vi "Lab Panel V5.24.1.vi"() -> ()   [LabVIEW 2013] (continued)
                n201 = Unbundle(w203) -> ("id1"=→"LAB01-TP":bool, "id2"=→"LAB02-TP":bool, "id3"=→"LAB03-TP":bool, "id4"=→"LAB04-TP":bool, "id5"=→"LAB05-TP":bool)
                n202 = local read "TEMP LA05"() -> (w211:T9)
                n203 = local read "TEMP LA04"() -> (w218:T9)
                n204 = local read "TEMP LA02"() -> (w232:T9)
                n205 = local read "TEMP LA03"() -> (w225:T9)
                n206 = local read "TEMP LA01"() -> (w239:T9)
                n207 = Bundle(cluster=w225, "TL-1"=w223, "TN-1"=w222, "TL-2"=w221, "TN-2"=w220) -> (w224:T9)  [unwired: 4 in]
                n208 = Bundle(cluster=w239, "TL-1"=w238, "TN-1"=w237, "TL-2"=w236, "TN-2"=w235) -> (w234:T9)  [unwired: 4 in]
                n209 = Bundle(cluster=w232, "TL-1"=w230, "TN-1"=w229, "TL-2"=w228, "TN-2"=w227) -> (w231:T9)  [unwired: 4 in]
                n210 = Bundle(cluster=w218, "TL-1"=w217, "TN-1"=w216, "TL-2"=w215, "TN-2"=w214) -> (w213:T9)  [unwired: 4 in]
                n211 = Bundle(cluster=w211, "TL-1"=w210, "TN-1"=w209, "TL-2"=w208, "TN-2"=w207) -> (w206:T9)  [unwired: 4 in]
                n212 = local write "TEMP LA03"(w224) -> ()
                n213 = local write "TEMP LA01"(w234) -> ()
                n214 = local write "TEMP LA02"(w231) -> ()
                n215 = local write "TEMP LA05"(w206) -> ()
                n216 = local write "TEMP LA04"(w213) -> ()
              }
            }
            frame #2 {
              w253 = 0
              n217 = local read "LAB01 TEMP"() -> (w255:T12)
              n218 = local read "SIG LAB01-2"() -> (w250:T2)
              n219 = Unbundle By Name(w255) -> ("T1 Live"=w248:dbl, "T1 Neut"=w247:dbl, "T2 Live"=w246:dbl, "T2 Neut"=w245:dbl)  [unwired: 2 out]
              n220 = local read "SIG LAB01-1"() -> (w252:T2)
              n221 = local read "TEMP LA01"() -> (w256:T9)
              n222 = Bundle By Name(cluster=w256, "TL-1"=w248, "TN-1"=w247, "TL-2"=w246, "TN-2"=w245, "TL -1COUNT"=w253, "TN-1 COUNT"=w253, "TL-2 COUNT"=w253, "TN-2 COUNT"=w253) -> (w254:T9)
              n223 = Bundle(cluster=w252, "Tmp Live"=w248, "Tmp Neut"=w247) -> (w251:T2)  [unwired: 3 in]
              n224 = Bundle(cluster=w250, "Tmp Live"=w246, "Tmp Neut"=w245) -> (w249:T2)  [unwired: 3 in]
              n225 = local write "SIG LAB01-2"(w249) -> ()
              n226 = local write "SIG LAB01-1"(w251) -> ()
              n227 = local write "TEMP LA01"(w254) -> ()
            }
            frame #3 {
              w265 = 0
              n228 = local read "LAB02 TEMP"() -> (w267:T12)
              n229 = Unbundle By Name(w267) -> ("T1 Live"=w260:dbl, "T1 Neut"=w259:dbl, "T2 Live"=w258:dbl, "T2 Neut"=w257:dbl)  [unwired: 2 out]
              n230 = local read "SIG LAB02-1"() -> (w264:T2)
              n231 = local read "SIG LAB02-2"() -> (w263:T2)
              n232 = local read "TEMP LA02"() -> (w268:T9)
              n233 = Bundle By Name(cluster=w268, "TL-1"=w260, "TN-1"=w259, "TL-2"=w258, "TN-2"=w257, "TL -1COUNT"=w265, "TN-1 COUNT"=w265, "TL-2 COUNT"=w265, "TN-2 COUNT"=w265) -> (w266:T9)
              n234 = Bundle(cluster=w263, "Tmp Live"=w258, "Tmp Neut"=w257) -> (w261:T2)  [unwired: 3 in]
              n235 = Bundle(cluster=w264, "Tmp Live"=w260, "Tmp Neut"=w259) -> (w262:T2)  [unwired: 3 in]
              n236 = local write "TEMP LA02"(w266) -> ()
              n237 = local write "SIG LAB02-1"(w262) -> ()
              n238 = local write "SIG LAB02-2"(w261) -> ()
            }
            frame #4 {
              w277 = 0
              n239 = local read "LAB03 TEMP"() -> (w279:T12)
              n240 = Unbundle By Name(w279) -> ("T1 Live"=w272:dbl, "T1 Neut"=w271:dbl, "T2 Live"=w270:dbl, "T2 Neut"=w269:dbl)  [unwired: 2 out]
              n241 = local read "SIG LAB03-1"() -> (w276:T2)
              n242 = local read "SIG LAB03-2"() -> (w275:T2)
              n243 = local read "TEMP LA03"() -> (w280:T9)
              n244 = Bundle By Name(cluster=w280, "TL-1"=w272, "TN-1"=w271, "TL-2"=w270, "TN-2"=w269, "TL -1COUNT"=w277, "TN-1 COUNT"=w277, "TL-2 COUNT"=w277, "TN-2 COUNT"=w277) -> (w278:T9)
              n245 = Bundle(cluster=w275, "Tmp Live"=w270, "Tmp Neut"=w269) -> (w273:T2)  [unwired: 3 in]
              n246 = Bundle(cluster=w276, "Tmp Live"=w272, "Tmp Neut"=w271) -> (w274:T2)  [unwired: 3 in]
              n247 = local write "TEMP LA03"(w278) -> ()
              n248 = local write "SIG LAB03-2"(w273) -> ()
              n249 = local write "SIG LAB03-1"(w274) -> ()
            }
            frame #5 {
              w289 = 0
              n250 = local read "LAB04 TEMP"() -> (w291:T12)
              n251 = Unbundle By Name(w291) -> ("T1 Live"=w284:dbl, "T1 Neut"=w283:dbl, "T2 Live"=w282:dbl, "T2 Neut"=w281:dbl)  [unwired: 2 out]
              n252 = local read "SIG LAB04-2"() -> (w287:T2)
              n253 = local read "SIG LAB04-1"() -> (w288:T2)
              n254 = local read "TEMP LA04"() -> (w292:T9)
              n255 = Bundle By Name(cluster=w292, "TL-1"=w284, "TN-1"=w283, "TL-2"=w282, "TN-2"=w281, "TL -1COUNT"=w289, "TN-1 COUNT"=w289, "TL-2 COUNT"=w289, "TN-2 COUNT"=w289) -> (w290:T9)
              n256 = Bundle(cluster=w287, "Tmp Live"=w282, "Tmp Neut"=w281) -> (w285:T2)  [unwired: 3 in]
              n257 = Bundle(cluster=w288, "Tmp Live"=w284, "Tmp Neut"=w283) -> (w286:T2)  [unwired: 3 in]
              n258 = local write "SIG LAB04-2"(w285) -> ()
              n259 = local write "TEMP LA04"(w290) -> ()
              n260 = local write "SIG LAB04-1"(w286) -> ()
            }
            frame #6 {
              w301 = 0
              n261 = local read "LAB05 TEMP"() -> (w303:T12)
              n262 = Unbundle By Name(w303) -> ("T1 Live"=w296:dbl, "T1 Neut"=w295:dbl, "T2 Live"=w294:dbl, "T2 Neut"=w293:dbl)  [unwired: 2 out]
              n263 = local read "SIG LAB05-2"() -> (w299:T2)
              n264 = local read "SIG LAB05-1"() -> (w300:T2)
              n265 = local read "TEMP LA05"() -> (w304:T9)
              n266 = Bundle By Name(cluster=w304, "TL-1"=w296, "TN-1"=w295, "TL-2"=w294, "TN-2"=w293, "TL -1COUNT"=w301, "TN-1 COUNT"=w301, "TL-2 COUNT"=w301, "TN-2 COUNT"=w301) -> (w302:T9)
              n267 = Bundle(cluster=w299, "Tmp Live"=w294, "Tmp Neut"=w293) -> (w297:T2)  [unwired: 3 in]
              n268 = Bundle(cluster=w300, "Tmp Live"=w296, "Tmp Neut"=w295) -> (w298:T2)  [unwired: 3 in]
              n269 = local write "SIG LAB05-2"(w297) -> ()
              n270 = local write "SIG LAB05-1"(w298) -> ()
              n271 = local write "TEMP LA05"(w302) -> ()
            }
          }
        }
        frame #9 {
          # "enable front panel, all settings done"
          n272 = property on="Tab Control 2" class="TabCtl (strict)"("DisabledEnum"=T16."Enabled" ("Disabled")) -> ()  [unwired: 2 in, 2 out]
          n273 = property on="Tab Control 2" class="TabCtl (strict)"("Value"=0) -> ()  [unwired: 2 in, 2 out]
        }
        frame #10 {
          n274 = property on="Tab Control 2" class="TabCtl (strict)"("Value"=0) -> ()  [unwired: 2 in, 2 out]
        }
      }
    }
    frame #2 {
      n275 = node-c288("loop  delay(mS)") -> (w310:T18)  [unwired: 3 in]
      n276 = timed-loop {
        timing: w310 -> [_]
        timing-out: [_] -> w309
        i -> [w336]
        stop <- w313 stop-if-true
        n277 = node-c288() -> ()  [unwired: 1 in, 1 out]
        n278 = local read "Resets Done"() -> (w315:dbl)
        n279 = Greater?(x=w315, y=50) -> (0:w311:bool)
        n280 = local read "SELECT LAB05-2"() -> (w316:T3)
        n281 = local read "SELECT LAB05-1"() -> (w317:T3)
        n282 = local read "SELECT LAB04-2"() -> (w318:T3)
        n283 = local read "SELECT LAB03-1"() -> (w321:T3)
        n284 = Or(x=w311, y="stop") -> (x .or. y?=w313:bool)
        n285 = local read "SELECT LAB02-2"() -> (w322:T3)
        n286 = local read "SELECT LAB01-1"() -> (w325:T3)
        n287 = local read "SELECT LAB03-2"() -> (w320:T3)
        n288 = local read "SELECT LAB01-2"() -> (w324:T3)
        n289 = local read "SELECT LAB04-1"() -> (w319:T3)
        n290 = local read "SELECT LAB02-1"() -> (w323:T3)
        n291 = local read "run lab03-2"() -> (w330:bool)
        n292 = local read "run lab04-1"() -> (w329:bool)
        n293 = local read "run lab05-1"() -> (w327:bool)
        n294 = local read "run lab04-2"() -> (w328:bool)
        n295 = local read "run lab05-2"() -> (w326:bool)
        n296 = local read "run lab03-1"() -> (w331:bool)
        n297 = local read "run lab02-2"() -> (w332:bool)
        n298 = local read "run lab02-1"() -> (w333:bool)
        n299 = local read "run lab01-1"() -> (w335:bool)
        n300 = local read "run lab01-2"() -> (w334:bool)
        n301 = global write "Global display 1.vi" "stop disp"(w313) -> ()
        n302 = stacked-sequence {
          seq-local: [_ w402 _ _ _ _ _ _ _ _ _ _ _ _ _ _ _ _ _ _ _ _ _ _] -> [_ _ _ _ _ w2503 _ _ _ _ _ _ _ _ _ _ _ _ _ _ _ _ _ _]
          seq-local: [_ w401 _ _ _ _ _ _ _ _ _ _ _ _ _ _ _ _ _ _ _ _ _ _] -> [_ _ _ _ _ w2502 _ _ _ _ _ _ _ _ _ _ _ _ _ _ _ _ _ _]
          seq-local: [_ w388 _ _ _ _ _ _ _ _ _ _ _ _ _ _ _ _ _ _ _ _ _ _] -> [_ _ _ _ _ w2501 _ _ _ _ _ _ _ _ _ _ _ _ _ _ _ _ _ _]
          seq-local: [_ w387 _ _ _ _ _ _ _ _ _ _ _ _ _ _ _ _ _ _ _ _ _ _] -> [_ _ _ _ _ w2500 _ _ _ _ _ _ _ _ _ _ _ _ _ _ _ _ _ _]
          seq-local: [_ w386 _ _ _ _ _ _ _ _ _ _ _ _ _ _ _ _ _ _ _ _ _ _] -> [_ _ _ _ _ w2499 _ _ _ _ _ _ _ _ _ _ _ _ _ _ _ _ _ _]
          seq-local: [_ w385 _ _ _ _ _ _ _ _ _ _ _ _ _ _ _ _ _ _ _ _ _ _] -> [_ _ _ _ _ w2498 _ _ _ _ _ _ _ _ _ _ _ _ _ _ _ _ _ _]
          seq-local: [_ w384 _ _ _ _ _ _ _ _ _ _ _ _ _ _ _ _ _ _ _ _ _ _] -> [_ _ _ _ _ w2497 _ _ _ _ _ _ _ _ _ _ _ _ _ _ _ _ _ _]
          seq-local: [_ w383 _ _ _ _ _ _ _ _ _ _ _ _ _ _ _ _ _ _ _ _ _ _] -> [_ _ _ _ _ w2496 _ _ _ _ _ _ _ _ _ _ _ _ _ _ _ _ _ _]
          seq-local: [_ w382 _ _ _ _ _ _ _ _ _ _ _ _ _ _ _ _ _ _ _ _ _ _] -> [_ _ _ _ _ w2495 _ _ _ _ _ _ _ _ _ _ _ _ _ _ _ _ _ _]
          seq-local: [_ w381 _ _ _ _ _ _ _ _ _ _ _ _ _ _ _ _ _ _ _ _ _ _] -> [_ _ _ _ _ w2494 _ _ _ _ _ _ _ _ _ _ _ _ _ _ _ _ _ _]
          seq-local: [_ _ _ _ _ _ _ _ _ _ _ w3626 _ _ _ _ _ _ _ _ _ _ _ _] -> [_ _ _ _ _ _ _ _ _ _ _ _ w3647 _ _ _ _ _ _ _ _ _ _ _]
          tunnel: w335 -> [_ _ w418 w666 w2093 w2523 w2838 w3325 _ _ _ _ _ w3929 _ w4886 _ _ w5173 w5476 w5657 _ _ _]
          tunnel: w334 -> [_ _ w417 w664 w2092 w2522 w2839 w3324 _ _ _ _ _ w3928 _ w4884 _ _ w5172 w5475 w5655 _ _ _]
          tunnel: w333 -> [_ _ w416 w662 w2091 w2521 w2837 w3323 _ _ _ _ _ w3927 _ w4882 _ _ w5171 w5474 w5654 _ _ _]
          tunnel: w332 -> [_ _ w415 w660 w2090 w2520 w2836 w3322 _ _ _ _ _ w3926 _ w4880 _ _ w5170 w5473 w5653 _ _ _]
          tunnel: w331 -> [_ _ w414 w658 w2089 w2519 w2835 w3321 _ _ _ _ _ w3925 _ w4878 _ _ w5169 w5472 w5652 _ _ _]
          tunnel: w330 -> [_ _ w413 w656 w2088 w2518 w2834 w3320 _ _ _ _ _ w3924 _ w4876 _ _ w5168 w5471 w5651 _ _ _]
          tunnel: w329 -> [_ _ w412 w654 w2087 w2517 w2833 w3319 _ _ _ _ _ w3923 _ w4874 _ _ w5167 w5470 w5650 _ _ _]
          tunnel: w328 -> [_ _ w411 w652 w2086 w2516 w2832 w3318 _ _ _ _ _ w3922 _ w4872 _ _ w5166 w5469 w5649 _ _ _]
          tunnel: w327 -> [_ _ w410 w650 w2085 w2515 w2831 w3317 _ _ _ _ _ w3921 _ w4870 _ _ w5165 w5468 w5648 _ _ _]
          tunnel: w326 -> [_ _ w409 w648 w2084 w2514 w2830 w3316 _ _ _ _ _ w3920 _ w4868 _ _ w5164 w5467 w5647 _ _ _]
          tunnel: w325 -> [_ _ _ w665 w2083 w2513 _ _ _ _ _ _ _ _ _ w4888 _ _ _ _ _ w6001 _ _]
          tunnel: w324 -> [_ _ _ w663 w2082 w2512 _ _ _ _ _ _ _ _ _ w4883 _ _ _ _ _ w6000 _ _]
          tunnel: w323 -> [_ _ _ w661 w2081 w2511 _ _ _ _ _ _ _ _ _ w4881 _ _ _ _ _ w5999 _ _]
          tunnel: w322 -> [_ _ _ w659 w2080 w2510 _ _ _ _ _ _ _ _ _ w4879 _ _ _ _ _ w5998 _ _]
          tunnel: w321 -> [_ _ _ w657 w2079 w2509 _ _ _ _ _ _ _ _ _ w4877 _ _ _ _ _ w5997 _ _]
          tunnel: w320 -> [_ _ _ w655 w2078 w2508 _ _ _ _ _ _ _ _ _ w4875 _ _ _ _ _ w5996 _ _]
          tunnel: w319 -> [_ _ _ w653 w2077 w2507 _ _ _ _ _ _ _ _ _ w4873 _ _ _ _ _ w5995 _ _]
          tunnel: w318 -> [_ _ _ w651 w2076 w2506 _ _ _ _ _ _ _ _ _ w4871 _ _ _ _ _ w5994 _ _]
          tunnel: w317 -> [_ _ _ w649 w2075 w2505 _ _ _ _ _ _ _ _ _ w4869 _ _ _ _ _ w5993 _ _]
          tunnel: w316 -> [_ _ _ w647 w2074 w2504 _ _ _ _ _ _ _ _ _ w4867 _ _ _ _ _ w5992 _ _]
          tunnel: w311 -> [_ _ _ _ _ _ _ _ _ _ _ _ _ _ _ _ _ _ _ _ _ _ _ w6053]
          frame #0 {
            w344 = FALSE
            w349 = 0.5
            # "set up cycle control"
            n303 = local read "jig cycle"() -> (w348:dbl)
            n304 = local read "Amps Fail level"() -> (w342:dbl)
            n305 = local read "Simulate"() -> (w339:bool)
            n306 = Divide(x="JIG ON TIME (S)", y=w349) -> (x/y=→"on loops":dbl)
            n307 = Divide(x="JIG OFF TIME (S)", y=w349) -> (x/y=→"off loops":dbl)
            n308 = Increment(x=w348) -> (x+1=w347:dbl)
            n309 = local write "Simulate IND"(w339) -> ()
            n310 = global write "Global display 3.vi" "Amps Fail"(w342) -> ()
            n311 = local write "TEMP"(w344) -> ()
            n312 = local write "AI"(w344) -> ()
            n313 = local read "Network Directory"() -> (w341:path)
            n314 = local write "jig cycle"(w347) -> ()
            n315 = call "sub vi - check network dir v2.vi"("PATH"=w341) -> ("error"=w340:bool)  [unwired: 10 in]
            n316 = local write "network error"(w340) -> ()
            n317 = global write "Global display 3.vi" "network drive"(w340) -> ()
            n318 = event shown="[1] \"ADMIN\": Value Change" {
              selector: _ -> [_ _]
              dyn-events: _ -> [_ _]
              timeout: 10 -> [_ _]
              event Timeout {
                n319 = event-data() -> ()  [unwired: 1 in, 3 out]
              }
              event "ADMIN": Value Change {
                n320 = event-data() -> ()  [unwired: 1 in, 6 out]
                n321 = stacked-sequence {
                  seq-local: [_ w353 _] -> [_ _ w354]
                  frame #0 {
                    n322 = global write "Global 1.vi" "password"("9949") -> ()
                  }
                  frame #1 {
                    n323 = call "sub vi - password 1.vi"() -> ("RESULT"=w353:bool)  [unwired: 11 in]
                  }
                  frame #2 {
                    w356 = FALSE
                    n324 = property on="Tab Control 2" class="TabCtl (strict)"() -> ("Pages"=w360:refnum<vi>[])  [unwired: 2 in, 2 out]
                    n325 = Select(t=TRUE, s=w354, f=w356) -> (s? t:f=w355:bool)
                    n326 = Index Array(array=w360, index=8) -> (element=w358:refnum<vi>)
                    n327 = property class="Page"(reference=w358, "PageVis"=w355) -> ()  [unwired: 1 in, 2 out]
                    n328 = local write "ADMIN"(w356) -> ()
                  }
                }
              }
            }
          }
          frame #1 {
            w398 = 60.0
            # "convert temperature rise minutes to cycles"
            n329 = local read "SET LAB05-2"() -> (w362:T5)
            n330 = local read "SET LAB05-1"() -> (w364:T5)
            n331 = local read "SET LAB04-2"() -> (w366:T5)
            n332 = local read "SET LAB01-1"() -> (w380:T5)
            n333 = local read "SET LAB01-2"() -> (w378:T5)
            n334 = local read "SET LAB02-2"() -> (w374:T5)
            n335 = local read "SET LAB04-1"() -> (w368:T5)
            n336 = local read "SET LAB03-1"() -> (w372:T5)
            n337 = local read "SET LAB03-2"() -> (w370:T5)
            n338 = local read "SET LAB02-1"() -> (w376:T5)
            n339 = local read "JIG OFF TIME (S)"() -> (w403:dbl)
            n340 = local read "JIG ON TIME (S)"() -> (w404:dbl)
            n341 = Unbundle(w362) -> ("T-RISE mins"=w361:dbl)  [unwired: 4 out]
            n342 = Unbundle(w364) -> ("T-RISE mins"=w363:dbl)  [unwired: 4 out]
            n343 = Unbundle(w380) -> ("T-RISE mins"=w379:dbl)  [unwired: 4 out]
            n344 = Unbundle(w366) -> ("T-RISE mins"=w365:dbl)  [unwired: 4 out]
            n345 = Unbundle(w378) -> ("T-RISE mins"=w377:dbl)  [unwired: 4 out]
            n346 = Unbundle(w376) -> ("T-RISE mins"=w375:dbl)  [unwired: 4 out]
            n347 = Unbundle(w368) -> ("T-RISE mins"=w367:dbl)  [unwired: 4 out]
            n348 = Unbundle(w374) -> ("T-RISE mins"=w373:dbl)  [unwired: 4 out]
            n349 = Unbundle(w370) -> ("T-RISE mins"=w369:dbl)  [unwired: 4 out]
            n350 = Unbundle(w372) -> ("T-RISE mins"=w371:dbl)  [unwired: 4 out]
            n351 = Add(x=w404, y=w403) -> (x+y=w397:dbl)
            n352 = Multiply(x=w398, y=w369) -> (x*y=w393:dbl)
            n353 = Multiply(x=w398, y=w367) -> (x*y=w392:dbl)
            n354 = Multiply(x=w398, y=w365) -> (x*y=w391:dbl)
            n355 = Multiply(x=w398, y=w363) -> (x*y=w390:dbl)
            n356 = Multiply(x=w398, y=w361) -> (x*y=w389:dbl)
            n357 = Multiply(x=w398, y=w377) -> (x*y=w399:dbl)
            n358 = Multiply(x=w398, y=w371) -> (x*y=w394:dbl)
            n359 = Multiply(x=w398, y=w379) -> (x*y=w400:dbl)
            n360 = Multiply(x=w398, y=w375) -> (x*y=w396:dbl)
            n361 = Multiply(x=w398, y=w373) -> (x*y=w395:dbl)
            n362 = Divide(x=w390, y=w397) -> (x/y=w382:dbl)
            n363 = Divide(x=w391, y=w397) -> (x/y=w383:dbl)
            n364 = Divide(x=w392, y=w397) -> (x/y=w384:dbl)
            n365 = Divide(x=w389, y=w397) -> (x/y=w381:dbl)
            n366 = Divide(x=w394, y=w397) -> (x/y=w386:dbl)
            n367 = Divide(x=w400, y=w397) -> (x/y=w402:dbl)
            n368 = Divide(x=w399, y=w397) -> (x/y=w401:dbl)
            n369 = Divide(x=w396, y=w397) -> (x/y=w388:dbl)
            n370 = Divide(x=w395, y=w397) -> (x/y=w387:dbl)
            n371 = Divide(x=w393, y=w397) -> (x/y=w385:dbl)
          }
          frame #2 {
            # "control cycle loops"
            n372 = local read "JIG OFF TIME (S)"() -> (w407:dbl)
            n373 = local read "JIG ON TIME (S)"() -> (w406:dbl)
            n374 = local read "jig cycle"() -> (w420:dbl)
            n375 = local read "on loops"() -> (w422:dbl)
            n376 = local read "off loops"() -> (w421:dbl)
            n377 = Add(x=w407, y=w406) -> (x+y=w405:dbl)
            n378 = Add(x=w422, y=w421) -> (x+y=w408:dbl)
            n379 = Greater Or Equal?(x=w420, y=w408) -> (x >= y?=w419:bool)
            n380 = case shown="True" w419 {
              tunnel: w418 -> [_ w456]
              tunnel: w417 -> [_ w455]
              tunnel: w416 -> [_ w454]
              tunnel: w415 -> [_ w453]
              tunnel: w414 -> [_ w452]
              tunnel: w413 -> [_ w451]
              tunnel: w412 -> [_ w450]
              tunnel: w411 -> [_ w449]
              tunnel: w410 -> [_ w448]
              tunnel: w409 -> [_ w447]
              tunnel: w405 -> [_ w446]
              frame False {
              }
              frame True {
                # "increment cycle value and convert cycles to minutes for temp rise"
                n381 = stacked-sequence {
                  frame #0 {
                    n382 = local read "Temp read loop"() -> (w459:dbl)
                    n383 = Increment(x=w459) -> (x+1=w458:dbl)
                    n384 = local write "Temp read loop"(w458) -> ()
                  }
                  frame #1 {
                    n385 = local read "Temp read loop"() -> (w460:dbl)
                    n386 = Greater?(x=w460, y=20) -> (0:w462:bool)
                    n387 = case shown="True" w462 {
                      frame False {
                      }
                      frame True {
                        n388 = local write "Temp read loop"(1) -> ()
                      }
                    }
                  }
                }
                n389 = local read "JIG RELAY CYCLES"() -> (w445:T8)
                n390 = local read "Temp read loop"() -> (→"Tp Up":dbl)
                n391 = Unbundle By Name(w445) -> ("LAB01-1"=w443:dbl, "LAB01-2"=w441:dbl, "LAB02-1"=w439:dbl, "LAB02-2"=w437:dbl, "LAB03-1"=w435:dbl, "LAB03-2"=w433:dbl, "LAB04-1"=w431:dbl, "LAB04-2"=w429:dbl, "LAB05-1"=w427:dbl, "LAB05-2"=w425:dbl)
                n392 = stacked-sequence {
                  tunnel: w456 -> [w474 _ _ _ _ _ _ _ _ _]
                  tunnel: w455 -> [_ w491 _ _ _ _ _ _ _ _]
                  tunnel: w454 -> [_ _ w508 _ _ _ _ _ _ _]
                  tunnel: w453 -> [_ _ _ w525 _ _ _ _ _ _]
                  tunnel: w452 -> [_ _ _ _ w542 _ _ _ _ _]
                  tunnel: w451 -> [_ _ _ _ _ w559 _ _ _ _]
                  tunnel: w450 -> [_ _ _ _ _ _ w576 _ _ _]
                  tunnel: w449 -> [_ _ _ _ _ _ _ w593 _ _]
                  tunnel: w448 -> [_ _ _ _ _ _ _ _ w610 _]
                  tunnel: w447 -> [_ _ _ _ _ _ _ _ _ w627]
                  tunnel: w446 -> [w471 w488 w505 w522 w539 w556 w573 w590 w607 w624]
                  tunnel: w443 -> [w465 _ _ _ _ _ _ _ _ _]
                  tunnel: [w464 _ _ _ _ _ _ _ _ _] -> w442
                  tunnel: w441 -> [_ w482 _ _ _ _ _ _ _ _]
                  tunnel: [_ w481 _ _ _ _ _ _ _ _] -> w440
                  tunnel: w439 -> [_ _ w499 _ _ _ _ _ _ _]
                  tunnel: [_ _ w498 _ _ _ _ _ _ _] -> w438
                  tunnel: w437 -> [_ _ _ w516 _ _ _ _ _ _]
                  tunnel: [_ _ _ w515 _ _ _ _ _ _] -> w436
                  tunnel: w435 -> [_ _ _ _ w533 _ _ _ _ _]
                  tunnel: [_ _ _ _ w532 _ _ _ _ _] -> w434
                  tunnel: w433 -> [_ _ _ _ _ w550 _ _ _ _]
                  tunnel: [_ _ _ _ _ w549 _ _ _ _] -> w432
                  tunnel: w431 -> [_ _ _ _ _ _ w567 _ _ _]
                  tunnel: [_ _ _ _ _ _ w566 _ _ _] -> w430
                  tunnel: w429 -> [_ _ _ _ _ _ _ w584 _ _]
                  tunnel: [_ _ _ _ _ _ _ w583 _ _] -> w428
                  tunnel: w427 -> [_ _ _ _ _ _ _ _ w601 _]
                  tunnel: [_ _ _ _ _ _ _ _ w600 _] -> w426
                  tunnel: w425 -> [_ _ _ _ _ _ _ _ _ w618]
                  tunnel: [_ _ _ _ _ _ _ _ _ w617] -> w424
                  frame #0 {
                    n393 = local read "DISP LAB01-1"() -> (w469:T4)
                    n394 = Unbundle(w469) -> ("CYCLE"=w470:dbl)  [unwired: 2 out]
                    n395 = case shown="True" w474 {
                      tunnel: w470 -> [w476 w480]
                      tunnel: [w476 w479] -> w468
                      tunnel: w465 -> [w475 w478]
                      tunnel: [w475 w477] -> w464
                      frame False {
                      }
                      frame True {
                        n396 = Increment(x=w478) -> (x+1=w477:dbl)
                        n397 = Increment(x=w480) -> (x+1=w479:dbl)
                      }
                    }
                    n398 = Multiply(x=w468, y=w471) -> (x*y=w472:dbl)
                    n399 = Divide(x=w472, y=60.0) -> (x/y=w467:dbl)
                    n400 = Bundle(cluster=w469, "CYCLE"=w468, "MINS"=w467) -> (w466:T4)  [unwired: 1 in]
                    n401 = local write "DISP LAB01-1"(w466) -> ()
                  }
                  frame #1 {
                    n402 = local read "DISP LAB01-2"() -> (w486:T4)
                    n403 = Unbundle(w486) -> ("CYCLE"=w487:dbl)  [unwired: 2 out]
                    n404 = case shown="True" w491 {
                      tunnel: w487 -> [w493 w497]
                      tunnel: [w493 w496] -> w484
                      tunnel: w482 -> [w492 w495]
                      tunnel: [w492 w494] -> w481
                      frame False {
                      }
                      frame True {
                        n405 = Increment(x=w495) -> (x+1=w494:dbl)
                        n406 = Increment(x=w497) -> (x+1=w496:dbl)
                      }
                    }
                    n407 = Multiply(x=w484, y=w488) -> (x*y=w489:dbl)
                    n408 = Divide(x=w489, y=60.0) -> (x/y=w483:dbl)
                    n409 = Bundle(cluster=w486, "CYCLE"=w484, "MINS"=w483) -> (w485:T4)  [unwired: 1 in]
                    n410 = local write "DISP LAB01-2"(w485) -> ()
                  }
                  frame #2 {
                    n411 = local read "DISP LAB02-1"() -> (w503:T4)
                    n412 = Unbundle(w503) -> ("CYCLE"=w504:dbl)  [unwired: 2 out]
                    n413 = case shown="True" w508 {
                      tunnel: [w510 w514] -> w501
                      tunnel: w504 -> [w510 w513]
                      tunnel: w499 -> [w509 w512]
                      tunnel: [w509 w511] -> w498
                      frame False {
                      }
                      frame True {
                        n414 = Increment(x=w512) -> (x+1=w511:dbl)
                        n415 = Increment(x=w513) -> (x+1=w514:dbl)
                      }
                    }
                    n416 = Multiply(x=w501, y=w505) -> (x*y=w506:dbl)
                    n417 = Divide(x=w506, y=60.0) -> (x/y=w500:dbl)
                    n418 = Bundle(cluster=w503, "CYCLE"=w501, "MINS"=w500) -> (w502:T4)  [unwired: 1 in]
                    n419 = local write "DISP LAB02-1"(w502) -> ()
                  }
                  frame #3 {
                    n420 = local read "DISP LAB02-2"() -> (w520:T4)
                    n421 = Unbundle(w520) -> ("CYCLE"=w521:dbl)  [unwired: 2 out]
                    n422 = case shown="True" w525 {
                      tunnel: [w527 w531] -> w519
                      tunnel: w521 -> [w527 w530]
                      tunnel: w516 -> [w526 w529]
                      tunnel: [w526 w528] -> w515
                      frame False {
                      }
                      frame True {
                        n423 = Increment(x=w529) -> (x+1=w528:dbl)
                        n424 = Increment(x=w530) -> (x+1=w531:dbl)
                      }
                    }
                    n425 = Multiply(x=w519, y=w522) -> (x*y=w523:dbl)
                    n426 = Divide(x=w523, y=60.0) -> (x/y=w518:dbl)
                    n427 = Bundle(cluster=w520, "CYCLE"=w519, "MINS"=w518) -> (w517:T4)  [unwired: 1 in]
                    n428 = local write "DISP LAB02-2"(w517) -> ()
                  }
                  frame #4 {
                    n429 = local read "DISP LAB03-1"() -> (w537:T4)
                    n430 = Unbundle(w537) -> ("CYCLE"=w538:dbl)  [unwired: 2 out]
                    n431 = case shown="True" w542 {
                      tunnel: [w544 w548] -> w534
                      tunnel: w538 -> [w544 w547]
                      tunnel: w533 -> [w543 w546]
                      tunnel: [w543 w545] -> w532
                      frame False {
                      }
                      frame True {
                        n432 = Increment(x=w546) -> (x+1=w545:dbl)
                        n433 = Increment(x=w547) -> (x+1=w548:dbl)
                      }
                    }
                    n434 = Multiply(x=w534, y=w539) -> (x*y=w540:dbl)
                    n435 = Divide(x=w540, y=60.0) -> (x/y=w535:dbl)
                    n436 = Bundle(cluster=w537, "CYCLE"=w534, "MINS"=w535) -> (w536:T4)  [unwired: 1 in]
                    n437 = local write "DISP LAB03-1"(w536) -> ()
                  }
                  frame #5 {
                    n438 = local read "DISP LAB03-2"() -> (w554:T4)
                    n439 = Unbundle(w554) -> ("CYCLE"=w555:dbl)  [unwired: 2 out]
                    n440 = case shown="True" w559 {
                      tunnel: [w561 w565] -> w553
                      tunnel: w555 -> [w561 w564]
                      tunnel: w550 -> [w560 w563]
                      tunnel: [w560 w562] -> w549
                      frame False {
                      }
                      frame True {
                        n441 = Increment(x=w563) -> (x+1=w562:dbl)
                        n442 = Increment(x=w564) -> (x+1=w565:dbl)
                      }
                    }
                    n443 = Multiply(x=w553, y=w556) -> (x*y=w557:dbl)
                    n444 = Divide(x=w557, y=60.0) -> (x/y=w552:dbl)
                    n445 = Bundle(cluster=w554, "CYCLE"=w553, "MINS"=w552) -> (w551:T4)  [unwired: 1 in]
                    n446 = local write "DISP LAB03-2"(w551) -> ()
                  }
                  frame #6 {
                    n447 = local read "DISP LAB04-1"() -> (w571:T4)
                    n448 = Unbundle(w571) -> ("CYCLE"=w572:dbl)  [unwired: 2 out]
                    n449 = case shown="True" w576 {
                      tunnel: [w578 w582] -> w569
                      tunnel: w572 -> [w578 w581]
                      tunnel: w567 -> [w577 w580]
                      tunnel: [w577 w579] -> w566
                      frame False {
                      }
                      frame True {
                        n450 = Increment(x=w580) -> (x+1=w579:dbl)
                        n451 = Increment(x=w581) -> (x+1=w582:dbl)
                      }
                    }
                    n452 = Multiply(x=w569, y=w573) -> (x*y=w574:dbl)
                    n453 = Divide(x=w574, y=60.0) -> (x/y=w568:dbl)
                    n454 = Bundle(cluster=w571, "CYCLE"=w569, "MINS"=w568) -> (w570:T4)  [unwired: 1 in]
                    n455 = local write "DISP LAB04-1"(w570) -> ()
                  }
                  frame #7 {
                    n456 = local read "DISP LAB04-2"() -> (w588:T4)
                    n457 = Unbundle(w588) -> ("CYCLE"=w589:dbl)  [unwired: 2 out]
                    n458 = case shown="True" w593 {
                      tunnel: [w595 w599] -> w586
                      tunnel: w589 -> [w595 w598]
                      tunnel: w584 -> [w594 w597]
                      tunnel: [w594 w596] -> w583
                      frame False {
                      }
                      frame True {
                        n459 = Increment(x=w597) -> (x+1=w596:dbl)
                        n460 = Increment(x=w598) -> (x+1=w599:dbl)
                      }
                    }
                    n461 = Multiply(x=w586, y=w590) -> (x*y=w592:dbl)
                    n462 = Divide(x=w592, y=60.0) -> (x/y=w585:dbl)
                    n463 = Bundle(cluster=w588, "CYCLE"=w586, "MINS"=w585) -> (w587:T4)  [unwired: 1 in]
                    n464 = local write "DISP LAB04-2"(w587) -> ()
                  }
                  frame #8 {
                    n465 = local read "DISP LAB05-1"() -> (w605:T4)
                    n466 = Unbundle(w605) -> ("CYCLE"=w606:dbl)  [unwired: 2 out]
                    n467 = case shown="True" w610 {
                      tunnel: [w612 w616] -> w603
                      tunnel: w606 -> [w612 w615]
                      tunnel: w601 -> [w611 w614]
                      tunnel: [w611 w613] -> w600
                      frame False {
                      }
                      frame True {
                        n468 = Increment(x=w614) -> (x+1=w613:dbl)
                        n469 = Increment(x=w615) -> (x+1=w616:dbl)
                      }
                    }
                    n470 = Multiply(x=w603, y=w607) -> (x*y=w608:dbl)
                    n471 = Divide(x=w608, y=60.0) -> (x/y=w602:dbl)
                    n472 = Bundle(cluster=w605, "CYCLE"=w603, "MINS"=w602) -> (w604:T4)  [unwired: 1 in]
                    n473 = local write "DISP LAB05-1"(w604) -> ()
                  }
                  frame #9 {
                    n474 = local read "DISP LAB05-2"() -> (w623:T4)
                    n475 = Unbundle(w623) -> ("CYCLE"=w622:dbl)  [unwired: 2 out]
                    n476 = case shown="True" w627 {
                      tunnel: [w629 w633] -> w621
                      tunnel: w622 -> [w629 w632]
                      tunnel: w618 -> [w628 w631]
                      tunnel: [w628 w630] -> w617
                      frame False {
                      }
                      frame True {
                        n477 = Increment(x=w631) -> (x+1=w630:dbl)
                        n478 = Increment(x=w632) -> (x+1=w633:dbl)
                      }
                    }
                    n479 = Multiply(x=w621, y=w624) -> (x*y=w625:dbl)
                    n480 = Divide(x=w625, y=60.0) -> (x/y=w620:dbl)
                    n481 = Bundle(cluster=w623, "CYCLE"=w621, "MINS"=w620) -> (w619:T4)  [unwired: 1 in]
                    n482 = local write "DISP LAB05-2"(w619) -> ()
                  }
                }
                n483 = local write "jig cycle"(0) -> ()
                n484 = Bundle By Name(cluster=w445, "LAB01-1"=w442, "LAB01-2"=w440, "LAB02-1"=w438, "LAB02-2"=w436, "LAB03-1"=w434, "LAB03-2"=w432, "LAB04-1"=w430, "LAB04-2"=w428, "LAB05-1"=w426, "LAB05-2"=w424) -> (w444:T8)
                n485 = local write "JIG RELAY CYCLES"(w444) -> ()
              }
            }
          }
          frame #3 {
            # "START & STOP test RUN switch change, start test if true and stop test if false"
            n486 = Get Date/Time In Seconds() -> (seconds since 1Jan1904=w645:timestamp)
            n487 = local read "C drive data root dir"() -> (w638:path)
            n488 = Format Date/Time String(time format string (%c)="%b\\%a%d", seconds (now)=w645) -> (date/time string=w669:string)  [unwired: 1 in]
            n489 = Format Date/Time String(time format string (%c)="%H%M", seconds (now)=w645) -> (date/time string=w667:string)  [unwired: 1 in]
            n490 = Format Date/Time String(time format string (%c)="LabPanel%Y", seconds (now)=w645) -> (date/time string=w644:string)  [unwired: 1 in]
            n491 = Path To String(path=w638) -> (string=w641:string)
            n492 = global write "Global 1.vi" "C drive root path"(w638) -> ()
            n493 = local read "Ref deg C"() -> (w634:dbl)
            n494 = Concatenate Strings(w641, "\\") -> (w639:string)
            n495 = event shown="[1] \"RUN LAB01-1\": Value Change" {
              selector: _ -> [_ _ _ _ _ _ _ _ _ _ _]
              dyn-events: _ -> [_ _ _ _ _ _ _ _ _ _ _]
              timeout: 10 -> [_ _ _ _ _ _ _ _ _ _ _]
              tunnel: w639 -> [_ w682 w822 w963 w1103 w1243 w1383 w1523 w1663 w1803 w1944]
              tunnel: w669 -> [_ w681 w821 w962 w1102 w1242 w1382 w1522 w1662 w1802 w1943]
              tunnel: w667 -> [_ w679 w820 w961 w1101 w1241 w1381 w1521 w1661 w1801 w1942]
              tunnel: w665 -> [_ w680 _ _ _ _ _ _ _ _ _]
              tunnel: w666 -> [_ _ _ _ _ _ _ _ _ _ _]
              tunnel: w664 -> [_ _ _ _ _ _ _ _ _ _ _]
              tunnel: w663 -> [_ _ w819 _ _ _ _ _ _ _ _]
              tunnel: w662 -> [_ _ _ _ _ _ _ _ _ _ _]
              tunnel: w661 -> [_ _ _ w960 _ _ _ _ _ _ _]
              tunnel: w660 -> [_ _ _ _ _ _ _ _ _ _ _]
              tunnel: w659 -> [_ _ _ _ w1100 _ _ _ _ _ _]
              tunnel: w658 -> [_ _ _ _ _ _ _ _ _ _ _]
              tunnel: w657 -> [_ _ _ _ _ w1240 _ _ _ _ _]
              tunnel: w656 -> [_ _ _ _ _ _ _ _ _ _ _]
              tunnel: w655 -> [_ _ _ _ _ _ w1380 _ _ _ _]
              tunnel: w654 -> [_ _ _ _ _ _ _ _ _ _ _]
              tunnel: w653 -> [_ _ _ _ _ _ _ w1520 _ _ _]
              tunnel: w652 -> [_ _ _ _ _ _ _ _ _ _ _]
              tunnel: w651 -> [_ _ _ _ _ _ _ _ w1660 _ _]
              tunnel: w650 -> [_ _ _ _ _ _ _ _ _ _ _]
              tunnel: w649 -> [_ _ _ _ _ _ _ _ _ w1800 _]
              tunnel: w648 -> [_ _ _ _ _ _ _ _ _ _ _]
              tunnel: w647 -> [_ _ _ _ _ _ _ _ _ _ w1941]
              tunnel: w644 -> [_ w678 w818 w959 w1099 w1239 w1379 w1519 w1659 w1799 w1940]
              tunnel: [_ w677 w817 w958 w1098 w1238 w1378 w1518 w1658 w1798 w1939] -> w642
              tunnel: "RESET CYCLES TO ZERO?" -> [_ w676 w815 w956 w1096 w1236 w1376 w1516 w1656 w1796 w1937]
              tunnel: "YES" -> [_ w675 w814 w955 w1095 w1235 w1375 w1515 w1655 w1795 w1936]
              tunnel: "NO" -> [_ w674 w813 w954 w1094 w1234 w1374 w1514 w1654 w1794 w1935]
              tunnel: w634 -> [_ w671 w812 w952 w1093 w1233 w1373 w1513 w1653 w1793 w1933]
              event Timeout {
                n496 = event-data() -> ()  [unwired: 1 in, 3 out]
              }
              event "RUN LAB01-1": Value Change {
                n497 = event-data() -> ("NewVal"=w672:bool)  [unwired: 1 in, 5 out]
                n498 = local read "SIG LAB01-1"() -> (w673:T2)
                n499 = local write "run lab01-1"(w672) -> ()
                n500 = case shown="True" w672 {
                  tunnel: w682 -> [_ w720]
                  tunnel: w681 -> [_ w719]
                  tunnel: w680 -> [w684 w718]
                  tunnel: w679 -> [_ w717]
                  tunnel: w678 -> [_ w716]
                  tunnel: [w683 w715] -> w677
                  tunnel: w676 -> [_ w714]
                  tunnel: w675 -> [_ w713]
                  tunnel: w674 -> [_ w712]
                  tunnel: w673 -> [_ w711]
                  tunnel: w671 -> [_ w710]
                  frame False {
                    # "stop test"
                    n501 = stacked-sequence {
                      tunnel: w684 -> [_ w696 _]
                      tunnel: [_ w688 _] -> w683
                      frame #0 {
                        n502 = local read "DISP LAB01-1"() -> (w687:T4)
                        n503 = Bundle(cluster=w687, "STATUS"="STOP") -> (w685:T4)  [unwired: 2 in]
                        n504 = local write "DISP LAB01-1"(w685) -> ()
                      }
                      frame #1 {
                        n505 = local read "DISP LAB01-1"() -> (w695:T4)
                        n506 = Unbundle(w695) -> ("CYCLE"=w693:dbl, "MINS"=w694:dbl)  [unwired: 1 out]
                        n507 = case shown="\"CYCLE TEST\"" w696 {
                          tunnel: w694 -> [_ _ w703]
                          tunnel: w693 -> [w701 w702 _]
                          tunnel: [w701 w702 w703] -> w692
                          frame "CHART TEST", Default {
                          }
                          frame "CYCLE TEST" {
                          }
                          frame "T-RISE TEST" {
                          }
                        }
                        n508 = local read "TDMS LAB01-1"() -> (w700:refnum<k34>)
                        n509 = Build Array("STOPPED") -> (w697:string[])
                        n510 = Build Array(w692) -> (w691:dbl[])
                        n511 = TDMS Write(0:w700, 5:"TEST RESULT", 7:w697, 9:w691) -> (4:w689:refnum<k34>, 15:w690:errorcluster)  [unwired: 2 in, 2 out]
                        n512 = TDMS Close(8:w690, 11:w689) -> (0:w688:errorcluster)  [unwired: 1 out]
                      }
                      frame #2 {
                        n513 = stacked-sequence {
                          tunnel: "LAB01-1" -> [w706 w708]
                          frame #0 {
                            n514 = call "sub vi - defrag tdms v1.vi"("panel id"=w706) -> ("error out"=w705:errorcluster)  [unwired: 10 in]
                            n515 = local write "data file error"(w705) -> ()
                          }
                          frame #1 {
                            n516 = call "Save data file (stop) v3.vi"("panel id"=w708) -> ("network file save error"=w707:errorcluster)  [unwired: 9 in, 1 out]
                            n517 = local write "RESULT LAB01-1"(FALSE) -> ()
                            n518 = local write "data file error"(w707) -> ()
                          }
                        }
                      }
                    }
                  }
                  frame True {
                    n519 = stacked-sequence {
                      seq-local: [w722 _] -> [_ w726]
                      tunnel: w720 -> [_ w736]
                      tunnel: w719 -> [_ w735]
                      tunnel: w718 -> [_ w734]
                      tunnel: w717 -> [_ w733]
                      tunnel: w716 -> [_ w732]
                      tunnel: [_ w731] -> w715
                      tunnel: w714 -> [_ w730]
                      tunnel: w713 -> [_ w729]
                      tunnel: w712 -> [_ w728]
                      tunnel: w711 -> [w724 w727]
                      tunnel: w710 -> [_ w725]
                      frame #0 {
                        n520 = Unbundle(w724) -> ("AMPS"=w723:dbl)  [unwired: 4 out]
                        n521 = call "Check For Amps on v1.vi"("ID"="LAB01-1", "amps"=w723) -> ("amps"=w722:bool)  [unwired: 9 in]
                      }
                      frame #1 {
                        n522 = case shown="True" w726 {
                          tunnel: w736 -> [_ w749]
                          tunnel: w735 -> [_ w748]
                          tunnel: w734 -> [_ w747]
                          tunnel: w733 -> [_ w746]
                          tunnel: w732 -> [_ w745]
                          tunnel: [errorcluster {"status"=FALSE, "code"=0, "source"=""} ("error out") w744] -> w731
                          tunnel: w730 -> [_ w743]
                          tunnel: w729 -> [_ w742]
                          tunnel: w728 -> [_ w741]
                          tunnel: w727 -> [_ w740]
                          tunnel: w725 -> [_ w739]
                          frame False {
                            w737 = FALSE
                            n523 = local write "RUN LAB01-1"(w737) -> ()
                            n524 = local write "run lab01-1"(w737) -> ()
                          }
                          frame True {
                            n525 = stacked-sequence {
                              seq-local: [w750 _ _ _ _] -> [_ w771 _ _ _]
                              tunnel: w749 -> [w755 _ _ _ _]
                              tunnel: w748 -> [w751 _ _ _ _]
                              tunnel: w747 -> [w765 _ _ _ _]
                              tunnel: w746 -> [w758 _ _ _ _]
                              tunnel: w745 -> [w753 _ _ _ _]
                              tunnel: [_ w772 _ _ _] -> w744
                              tunnel: w743 -> [_ _ _ w793 _]
                              tunnel: w742 -> [_ _ _ w803 _]
                              tunnel: w741 -> [_ _ _ w802 _]
                              tunnel: w740 -> [_ _ _ _ _]
                              tunnel: w739 -> [_ _ _ _ w809]
                              frame #0 {
                                w752 = "\\"
                                n526 = case shown="\"CHART TEST\", Default" w765 {
                                tunnel: ["L01-1-CHART TEST-" "L01-1-CYCLE TEST-" "L01-1-T-RISE TEST-"] -> w761
                                frame "CHART TEST", Default {
                                }
                                frame "CYCLE TEST" {
                                }
                                frame "T-RISE TEST" {
                                }
                                }
                                n527 = local read "SET LAB01-1"() -> (w760:T5)
                                n528 = Unbundle(w760) -> ("DESCRIPTION"=w759:string)  [unwired: 4 out]
                                n529 = Concatenate Strings(w755, "\\", w753, w752, w751, w752) -> (w762:string)
                                n530 = String To Path(string=w762) -> (path=w764:path)
                                n531 = Concatenate Strings(w762, w761, w759, "-", w758, ".tdms") -> (w750:string)
                                n532 = Create Folder(path (use dialog)=w764) -> (error out=w763:errorcluster)  [unwired: 2 in, 2 out]
                                n533 = call <vilib>:"Clear Errors.vi"("error in (no error)"=w763) -> ()  [unwired: 6 in, 1 out]
                                n534 = global write "Global 1.vi" "LAB01-1 FILE"(w750) -> ()
                              }
                              frame #1 {
                                (unwired) FALSE
                                n535 = String To Path(string=w771) -> (path=w769:path)
                                n536 = TDMS Open(6:FALSE, 10:T21."create or replace" ("operation (0:open)"), 11:w769) -> (0:w772:errorcluster, 3:→"TDMS LAB01-1":refnum<k34>)  [unwired: 4 in]
                              }
                              frame #2 {
                                n537 = local read "TDMS LAB01-1"() -> (w791:refnum<k34>)
                                n538 = local read "SET LAB01-1"() -> (w780:T5)
                                n539 = Build Array("Testers Name", "Description", "Set Test Cycles", "T-Rise minutes", "T-Rise Deg C") -> (w781:string[])
                                n540 = Unbundle(w780) -> ("NAME"=w779:string, "DESCRIPTION"=w778:string, "CYCLES"=w777:dbl, "T-RISE mins"=w776:dbl, "T-RISE deg C"=w775:dbl)
                                n541 = Number To Decimal String(number=w777) -> (decimal integer string=w790:string)  [unwired: 1 in]
                                n542 = Number To Decimal String(number=w776) -> (decimal integer string=w789:string)  [unwired: 1 in]
                                n543 = Number To Decimal String(number=w775) -> (decimal integer string=w788:string)  [unwired: 1 in]
                                n544 = Build Array(w779, w778, w790, w789, w788) -> (w787:string[])
                                n545 = TDMS Set Properties(5:w787, 7:w781, 11:w791) -> ()  [unwired: 3 in, 4 out]
                              }
                              frame #3 {
                                n546 = local read "DISP LAB01-1"() -> (w801:T4)
                                n547 = Concatenate Strings("LAB01-1  ", w793) -> (w792:string)
                                n548 = Two Button Dialog(message=w792, 1:w802, 2:w803) -> (T button?=w795:bool)
                                n549 = case shown="True" w795 {
                                tunnel: w801 -> [w806 w807]
                                tunnel: [w806 w807] -> w800
                                tunnel: [w805 w808] -> w799
                                tunnel: [w804 w808] -> w798
                                frame False {
                                n550 = Unbundle(w806) -> ("CYCLE"=w805:dbl, "MINS"=w804:dbl)  [unwired: 1 out]
                                }
                                frame True {
                                w808 = 0.0
                                }
                                }
                                n551 = Bundle(cluster=w800, "CYCLE"=w799, "MINS"=w798, "STATUS"="RUN") -> (w797:T4)
                                n552 = local write "DISP LAB01-1"(w797) -> ()
                              }
                              frame #4 {
                                n553 = local read "TEMP START LAB01-1"() -> (w811:cluster{"TL":dbl, "TN":dbl})
                                n554 = Bundle(cluster=w811, "TL"=w809, "TN"=w809) -> (w810:cluster{"TL":dbl, "TN":dbl})
                                n555 = local write "TEMP START LAB01-1"(w810) -> ()
                              }
                            }
                          }
                        }
                      }
                    }
                  }
                }
              }
              event "RUN LAB01-2": Value Change {
                n556 = event-data() -> ("NewVal"=w816:bool)  [unwired: 1 in, 5 out]
                n557 = local write "run lab01-2"(w816) -> ()
                n558 = case shown="True" w816 {
                  tunnel: w822 -> [_ w860]
                  tunnel: w821 -> [_ w859]
                  tunnel: w819 -> [w824 w858]
                  tunnel: w820 -> [_ w857]
                  tunnel: w818 -> [_ w856]
                  tunnel: [w823 w855] -> w817
                  tunnel: w815 -> [_ w854]
                  tunnel: w814 -> [_ w853]
                  tunnel: w813 -> [_ w852]
                  tunnel: w812 -> [_ w850]
                  frame False {
                    # "stop test"
                    n559 = stacked-sequence {
                      tunnel: w824 -> [w833 _]
                      tunnel: [w825 _] -> w823
                      frame #0 {
                        n560 = local read "DISP LAB01-2"() -> (w832:T4)
                        n561 = Unbundle(w832) -> ("CYCLE"=w830:dbl, "MINS"=w831:dbl)  [unwired: 1 out]
                        n562 = case shown="\"CHART TEST\", Default" w833 {
                          tunnel: w831 -> [_ _ w840]
                          tunnel: w830 -> [w838 w839 _]
                          tunnel: [w838 w839 w840] -> w829
                          frame "CHART TEST", Default {
                          }
                          frame "CYCLE TEST" {
                          }
                          frame "T-RISE TEST" {
                          }
                        }
                        n563 = local read "TDMS LAB01-2"() -> (w837:refnum<k34>)
                        n564 = Build Array("STOPPED") -> (w834:string[])
                        n565 = Build Array(w829) -> (w828:dbl[])
                        n566 = TDMS Write(0:w837, 5:"TEST RESULT", 7:w834, 9:w828) -> (4:w826:refnum<k34>, 15:w827:errorcluster)  [unwired: 2 in, 2 out]
                        n567 = TDMS Close(8:w827, 11:w826) -> (0:w825:errorcluster)  [unwired: 1 out]
                      }
                      frame #1 {
                        n568 = local read "DISP LAB01-2"() -> (w844:T4)
                        n569 = stacked-sequence {
                          tunnel: "LAB01-2" -> [w846 w848]
                          frame #0 {
                            n570 = call "sub vi - defrag tdms v1.vi"("panel id"=w846) -> ("error out"=w845:errorcluster)  [unwired: 10 in]
                            n571 = local write "data file error"(w845) -> ()
                          }
                          frame #1 {
                            n572 = call "Save data file (stop) v3.vi"("panel id"=w848) -> ("network file save error"=w847:errorcluster)  [unwired: 9 in, 1 out]
                            n573 = local write "RESULT LAB01-2"(FALSE) -> ()
                            n574 = local write "data file error"(w847) -> ()
                          }
                        }
                        n575 = Bundle(cluster=w844, "STATUS"="STOP") -> (w842:T4)  [unwired: 2 in]
                        n576 = local write "DISP LAB01-2"(w842) -> ()
                      }
                    }
                  }
                  frame True {
                    n577 = local read "SIG LAB01-2"() -> (w851:T2)
                    n578 = stacked-sequence {
                      seq-local: [w862 _] -> [_ w866]
                      tunnel: w860 -> [_ w876]
                      tunnel: w859 -> [_ w875]
                      tunnel: w858 -> [_ w874]
                      tunnel: w857 -> [_ w873]
                      tunnel: w856 -> [_ w872]
                      tunnel: [_ w871] -> w855
                      tunnel: w854 -> [_ w870]
                      tunnel: w853 -> [_ w869]
                      tunnel: w852 -> [_ w868]
                      tunnel: w851 -> [w861 w867]
                      tunnel: w850 -> [_ w865]
                      frame #0 {
                        n579 = Unbundle(w861) -> ("AMPS"=w864:dbl)  [unwired: 4 out]
                        n580 = call "Check For Amps on v1.vi"("ID"="LAB01-2", "amps"=w864) -> ("amps"=w862:bool)  [unwired: 9 in]
                      }
                      frame #1 {
                        n581 = case shown="True" w866 {
                          tunnel: w876 -> [_ w889]
                          tunnel: w875 -> [_ w888]
                          tunnel: w874 -> [_ w887]
                          tunnel: w873 -> [_ w886]
                          tunnel: w872 -> [_ w885]
